vi "connect_objects.vi"(8 "to object terminal index":i32, 9 "to object id":string, 10 "from object terminal index":i32, 11 "from object id":string) -> (0 "error out":errorcluster)   [LabVIEW 2020]
doc: "Connects two terminals of two objects with a wire on the block diagram of a labview vi. To get a new VI use \"new vi\" to add objects to a vi use \"add object\". If a frontpanel control/indicator reference is passed to this function, it will automatically use the corresponding terminal on the block diagram for wiring. Use get_object_terminals before wiring to find out which terminals to wire."
uses:
  G-AI Core/G-AI Core.lvlib
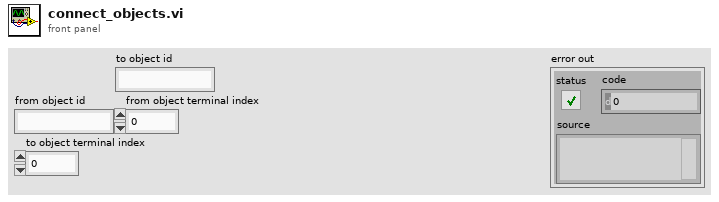
[diagram p1: front panel]
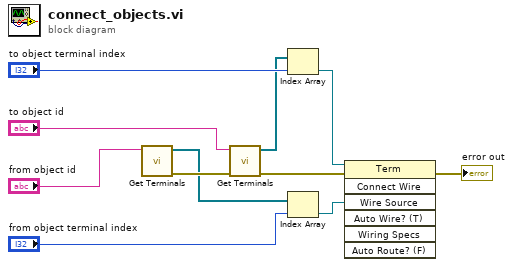
[diagram p0: block diagram]
diagram:
  n1 = call "Get Terminals.vi"("id"="from object id") -> ("error out"=w6:errorcluster, "Terminals"=w4:refnum<vi>[])  [unwired: 9 in]
  n2 = call "Get Terminals.vi"("error in"=w6, "id"="to object id") -> ("error out"=w3:errorcluster, "Terminals"=w1:refnum<vi>[])  [unwired: 8 in]
  n3 = Index Array(array=w1, index="to object terminal index") -> (element=w9:refnum<vi>)
  n4 = Index Array(array=w4, index="from object terminal index") -> (element=w8:refnum<vi>)
  n5 = invoke class="Term" method="Connect Wire"(reference=w9, error in=w3, "Wire Source"=w8) -> (error out=→"error out":errorcluster)  [unwired: 4 in, 6 out]
